vi "Generate Start Omega Measurement Command.vi"(0 "Sensor Address In":string="a", 1 "Sensor On/Off":bool, 7 "Measurement Type In (Normal)":i32(ring) items=["Normal", "Concurrent", "Continuous"], 11 "Error In (No Error)":errorcluster) -> (4 "Command":string, 15 "Error Out":errorcluster)   [LabVIEW 2015]
doc: "Generates a Normal or Concurrent Start Measurement Command, depending on the settings passed to the controls.\n\nStart Measurement aM!\nStart Measurement and Request CRC aMC!\nAdditional Measurements aM1! through aM9!\nAdditional Measurements and Request CRC aMC1! through aMC9!\nStart Concurrent Measurement aC!\nStart Concurrent Measurement and Request CRC aCC!\nAdditional Concurrent Measurements aC1! through aC9!\nAdditional Concurrent Measurements and Request CRC aCC1! through aCC9!\n\n\nNOTE: Continuous Measurements are continuously acquiring data, and should not be sent a Start Measurement Command."
uses:
  SDI-12.lvlib
panel:
  in  "Secondary Command":string="a"
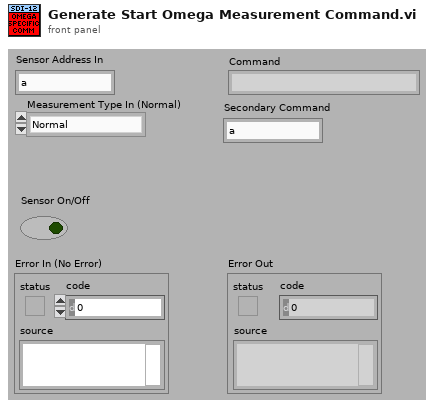
[diagram p1: front panel]
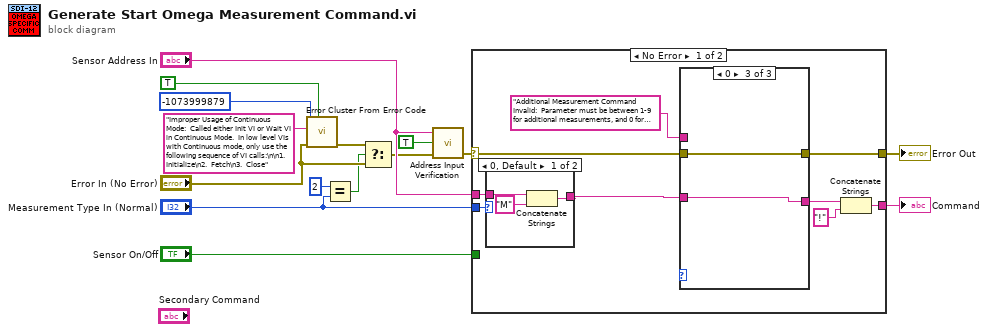
[diagram p0: block diagram]
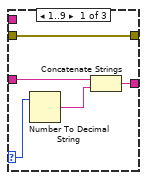
[diagram p2: hidden frame]
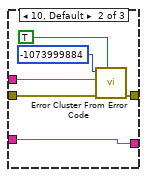
[diagram p3: hidden frame]
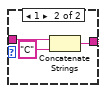
[diagram p4: hidden frame]
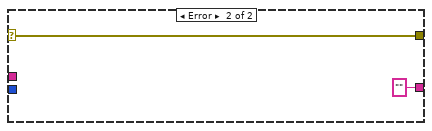
[diagram p5: hidden frame]
diagram:
  n1 = call <vilib>:"Error Cluster From Error Code.vi"("show call chain? (False)"=TRUE ("Error?"), "error in (no error)"="Error In (No Error)", "error message (\"\")"="Improper Usage of Continuous Mode:  Called either Init VI or Wait VI in Continuous Mode.  In low level VIs with Continuous mode, only use the following sequence of VI calls:\n\n1.  Initialize\n2.  Fetch\n3.  Close" ("error message (\"\")"), "error code (0)"=-1073999879 ("error code")) -> ("error out"=w7:errorcluster)  [unwired: 5 in]
  n2 = Equal?(x=2, y="Measurement Type In (Normal)") -> (x = y?=w1:bool)
  n3 = Select(t=w7, s=w1, f="Error In (No Error)") -> (s? t:f=w4:errorcluster)
  n4 = call "Address Input Verification.vi"("Error In (No Error)"=w4, "Error if Bad? (True)"=TRUE ("error if bad? (True)"), "Sensor Address In (a)"="Sensor Address In") -> ("Error Out"=w13:errorcluster)  [unwired: 1 in, 1 out]
  n5 = case shown="No Error" w13 {
    selector: w13 -> [w18 w46]
    tunnel: "Sensor Address In" -> [w25 _]
    tunnel: [w17 w46] -> w15
    tunnel: "Measurement Type In (Normal)" -> [w21 _]
    tunnel: "Sensor On/Off" -> [w20 _]
    tunnel: [w19 ""] -> w12
    frame No Error {
      n6 = case shown="0, Default" w21 {
        tunnel: w25 -> [w40 w44]
        tunnel: [w39 w42] -> w24
        frame 0, Default {
          n7 = Concatenate Strings(w40, "M" ("string")) -> (w39:string)
        }
        frame 1 {
          n8 = Concatenate Strings(w44, "C" ("string")) -> (w42:string)
        }
      }
      n9 = case shown="0" {
        selector: _ -> [w30 _ _]
        tunnel: w24 -> [w28 w34 w38]
        tunnel: [w27 w34 w38] -> w23
        tunnel: w18 -> [w26 w33 w37]
        tunnel: [w26 w32 w37] -> w17
        tunnel: "Additional Measurement Command Invalid:  Parameter must be between 1-9 for additional measurements, and 0 for default measurements. " ("error message (\"\")") -> [_ w31 _]
        frame 1..9 {
          n10 = Number To Decimal String(number=w30) -> (decimal integer string=w29:string)  [unwired: 1 in]
          n11 = Concatenate Strings(w28, w29) -> (w27:string)
        }
        frame 10, Default {
          n12 = call <vilib>:"Error Cluster From Error Code.vi"("show call chain? (False)"=TRUE, "error in (no error)"=w33, "error message (\"\")"=w31, "error code (0)"=-1073999884 ("error code")) -> ("error out"=w32:errorcluster)  [unwired: 5 in]
        }
        frame 0 {
        }
      }
      n13 = Concatenate Strings(w23, "!" ("string")) -> (w19:string)
    }
    frame Error {
    }
  }
  "Error Out" <- w15
  "Command" <- w12
